vi "median.vi"(11 "Array":dbl[](array[numeric])) -> (2 "s":dbl, 3 "m":dbl)   [LabVIEW 2014]
uses:
  <vilib>/Analysis/NI_AALBase.lvlib
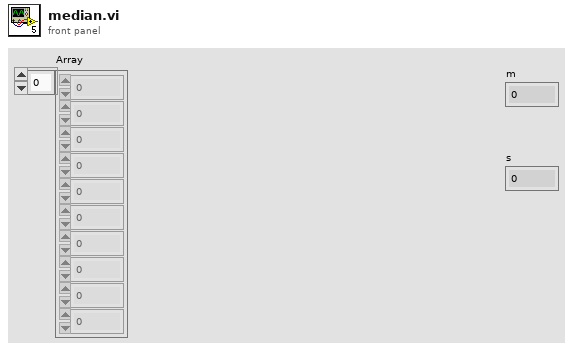
[diagram p1: front panel]
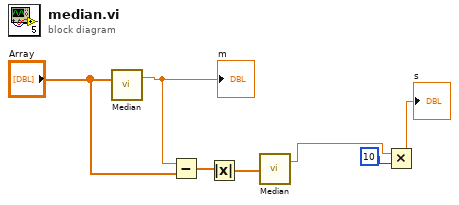
[diagram p0: block diagram]
diagram:
  n1 = call <vilib>:"Median.vi"("X"="Array") -> ("median"=w7:dbl)  [unwired: 1 out]
  "m" <- w7
  n2 = Subtract(x=w7, y="Array") -> (x-y=w5:dbl[])
  n3 = Absolute Value(x=w5) -> (abs(x)=w4:dbl[])
  n4 = call <vilib>:"Median.vi"("X"=w4) -> ("median"=w3:dbl)  [unwired: 1 out]
  n5 = Multiply(x=w3, y=10) -> (x*y=→"s":dbl)
